vi "Write Meta Data.vi"(6 "Meta Data":string, 11 "Linked List Definition in":refnum<class "Linked List Definition.lvclass">) -> (3 "Linked List Definition out":refnum<class "Linked List Definition.lvclass">)   [LabVIEW 2017, in "Linked Lists.lvlib" / "Linked List Definition.lvclass"]
uses:
  <vilib>/gpm_packages/@cs/linked-list/Source/Linked List/Linked List Definition/Linked List Definition.lvclass
  <vilib>/gpm_packages/@cs/linked-list/Source/Linked List/Linked List Definition/Linked List Definition.lvclass/Linked List Definition.ctl
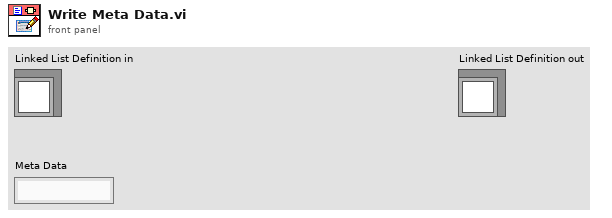
[diagram p1: front panel]
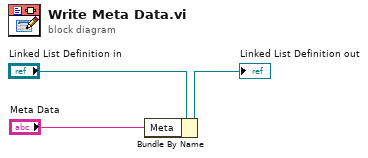
[diagram p0: block diagram]
diagram:
  n1 = Bundle By Name(cluster="Linked List Definition in", "Meta"="Meta Data") -> (→"Linked List Definition out":refnum<class "Linked List Definition.lvclass">)
